vi "Clamp AET Min_Vertical_shan.vi"(0 "Image":T4, 1 "Scanning axis":u16(ring)=1 items=["Left To Right", "Right To Left", "Top To Bottom", "Bottom To Top"], 5 "ROI Descriptor":T5 {"Contours"."Type" items=["No Selection", "Point", "Line", "Rectangle", "Oval", "Polygon", "Freehand Region", "Annulus", "Unused2", "Unused3", "Broken Line", "Freehand Line", "Rotated Rectangle"]}, 7 "Calibrated Image":T4, 9 "Coordinate System":T11 {"Measurement System"."Axis Reference" items=["Direct", "Indirect"]; "Measurement System"."Angle (deg)" format="%.2f"; "Measurement System"."Origin"."Y" format="%.2f"; "Measurement System"."Origin"."X" format="%.2f"; "Reference System"."Axis Reference" items=["Direct", "Indirect"]; "Reference System"."Angle (deg)" format="%.2f"; "Reference System"."Origin"."Y" format="%.2f"; "Reference System"."Origin"."X" format="%.2f"}, 11 "error in (no error)":errorcluster, 12 "Edge Options":T8={"Edge Polarity"=0, "Kernel Size"=3, "Width"=3, "Minimum Edge Strength"=10.0, "Interpolation Type"=enum."Bilinear Fixed", "Data Processing Method"=enum."Average"} {"Edge Polarity" items=["All Edges", "Rising Edges", "Falling Edges"]; "Minimum Edge Strength" format="%.2f"; "Width" step=2; "Kernel Size" step=2}) -> (3 "Edge Coordinates":cluster{"X":sgl, "Y":sgl}[](array[cluster]) {"Y" format="%.2f"; "X" format="%.2f"}, 6 "Distance":sgl format="%.2f", 8 "Coordinate System (duplicate)":T11 {"Measurement System"."Axis Reference" items=["Direct", "Indirect"]; "Measurement System"."Angle (deg)" format="%.2f"; "Measurement System"."Origin"."Y" format="%.2f"; "Measurement System"."Origin"."X" format="%.2f"; "Reference System"."Axis Reference" items=["Direct", "Indirect"]; "Reference System"."Angle (deg)" format="%.2f"; "Reference System"."Origin"."Y" format="%.2f"; "Reference System"."Origin"."X" format="%.2f"}, 10 "Search Lines":T1[](array[typedef]) {"Edge Info"."Distance (Real-World)" format="%.2f"; "Edge Info"."Location (Real-World)"."Y" format="%.2g"; "Edge Info"."Location (Real-World)"."X" format="%.2f"; "Edge Info"."Noise" format="%.2f"; "Edge Info"."Location (Pixel)"."Y" format="%.2g"; "Edge Info"."Location (Pixel)"."X" format="%.2f"; "Edge Info"."Strength" format="%.2f"; "Edge Info"."Distance (Pixel)" format="%.2f"}, 13 "Overlay Cluster out":T3 {"Search Lines"."Edge Info"."Distance (Real-World)" format="%.2f"; "Search Lines"."Edge Info"."Location (Real-World)"."Y" format="%.2g"; "Search Lines"."Edge Info"."Location (Real-World)"."X" format="%.2f"; "Search Lines"."Edge Info"."Noise" format="%.2f"; "Search Lines"."Edge Info"."Location (Pixel)"."Y" format="%.2g"; "Search Lines"."Edge Info"."Location (Pixel)"."X" format="%.2f"; "Search Lines"."Edge Info"."Strength" format="%.2f"; "Search Lines"."Edge Info"."Distance (Pixel)" format="%.2f"}, 14 "Perpendicular Lines":T6(array[cluster])=[{{"X"=55.0, "Y"=48.0}, {"X"=263.0, "Y"=104.0}}, {{"X"=53.0, "Y"=53.0}, {"X"=262.0, "Y"=109.0}}, {{"X"=52.0, "Y"=58.0}, {"X"=261.0, "Y"=113.0}}, {{"X"=51.0, "Y"=62.0}, {"X"=259.0, "Y"=118.0}}, {{"X"=49.0, "Y"=67.0}, {"X"=258.0, "Y"=123.0}}, {{"X"=48.0, "Y"=72.0}, {"X"=257.0, "Y"=128.0}}, {{"X"=47.0, "Y"=77.0}, {"X"=255.0, "Y"=133.0}}, {{"X"=46.0, "Y"=82.0}, {"X"=254.0, "Y"=138.0}}, {{"X"=44.0, "Y"=87.0}, {"X"=253.0, "Y"=142.0}}, {{"X"=43.0, "Y"=91.0}, {"X"=252.0, "Y"=147.0}}, {{"X"=42.0, "Y"=96.0}, {"X"=250.0, "Y"=152.0}}] {"?"."Y" format="%.2f"; "?"."X" format="%.2f"; "?"."Y" format="%.2f"; "?"."X" format="%.2f"}, 15 "error out":errorcluster)   [LabVIEW 2019, in "Algorithm.lvclass"]
doc: "Modified NI Vertical Max Clamp with Rake-3 which uses Advanced Edge Detection."
uses:
  FrameworkOverrides/Algorithm.lvclass
  <vilib>/vision/NI_Vision_Development_Module.lvlib
  <vilib>/vision/Measure.llb/Edge New.ctl
  <vilib>/vision/Measure.llb/Search Line.ctl
  <vilib>/vision/Image Controls.llb/IMAQ Image.ctl
  <vilib>/vision/Measure.llb/Edge Polarity.ctl
  <vilib>/vision/Measure.llb/Edge Options.ctl
panel:
  in  "Rect for the clamp":T7 {"Rotation" format="%.2f"; "Left" scale=0.0..1024.0; "Right" scale=0.0..1024.0}
  in  "Settings":T10={"Contrast"=50, "Filter width"=4, "Steepness"=2, "Subsampling Ratio"=5, "Show Search Area"=FALSE, "Show Search Lines"=FALSE, "Show Edges Found"=FALSE, "Show Result"=TRUE}
  out "Elapsed time (ms)":u32
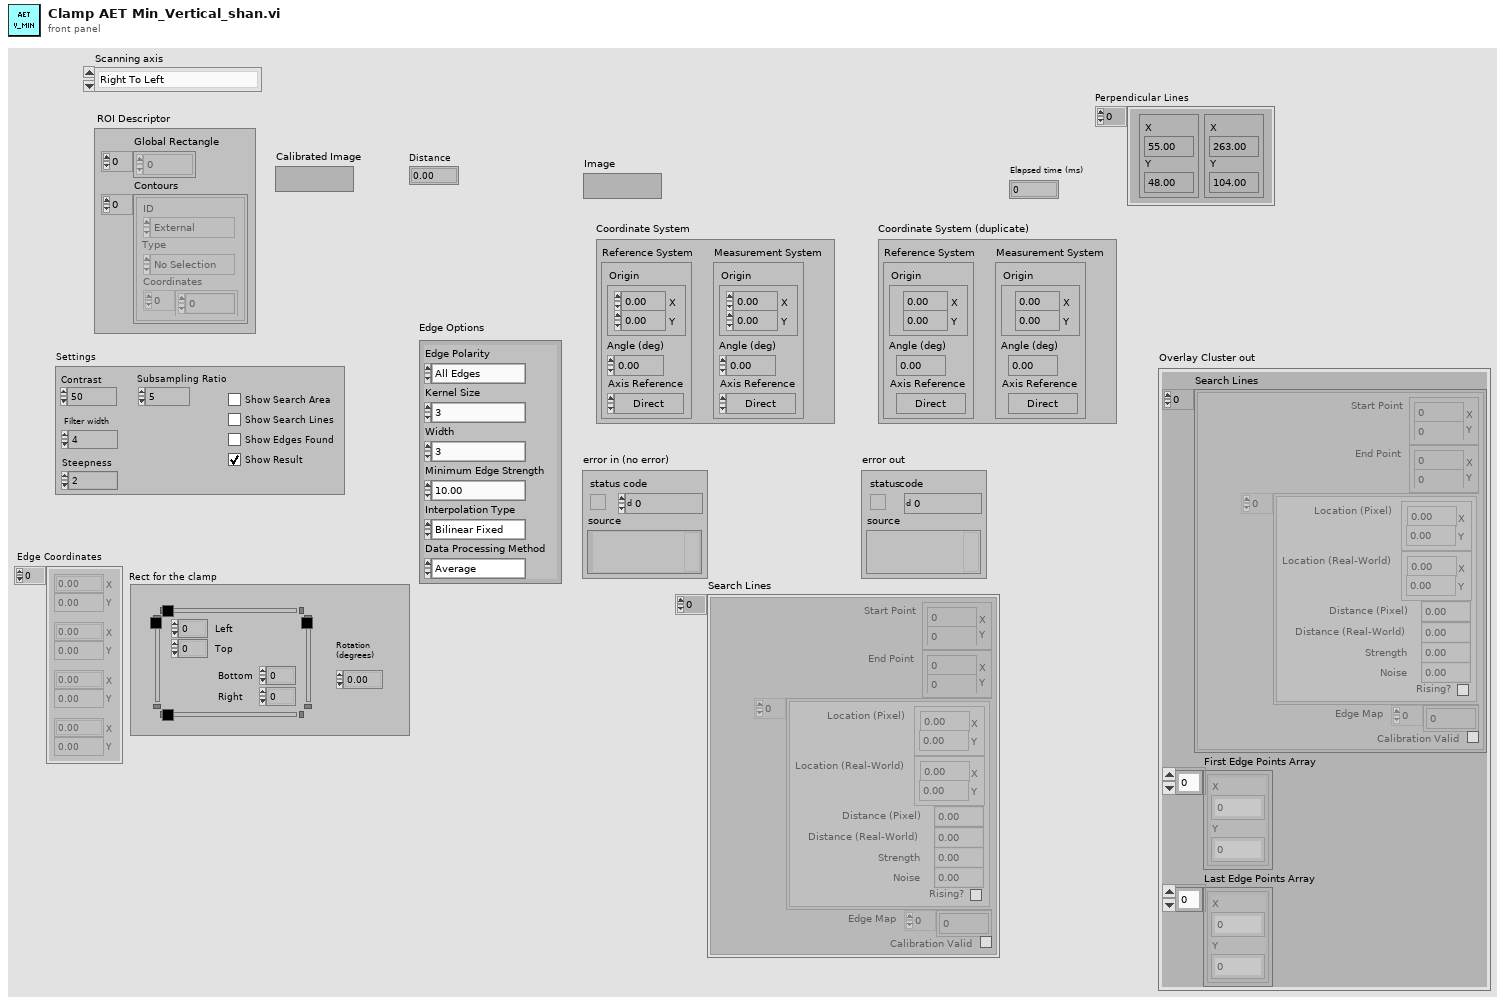
[diagram p1: front panel]
types:
  T1 = typedef "Search Line.ctl" = cluster{"Start Point":cluster{"X":sgl, "Y":sgl}, "End Point":cluster{"X":sgl, "Y":sgl}, "Edge Info":T2[], "Edge Map":dbl[], "Calibration Valid":bool}
  T2 = typedef "Edge New.ctl" = cluster{"Location (Pixel)":cluster{"X":sgl, "Y":sgl}, "Location (Real-World)":cluster{"X":sgl, "Y":sgl}, "Distance (Pixel)":dbl, "Distance (Real-World)":dbl, "Strength":dbl, "Noise":dbl, "Rising?":bool}
  T3 = cluster{"Search Lines":T1[], "First Edge Points Array":cluster{"X":sgl, "Y":sgl}[], "Last Edge Points Array":cluster{"X":sgl, "Y":sgl}[]}
  T4 = typedef "IMAQ Image.ctl" = refnum<image>
  T5 = typedef "ROI Descriptor" = cluster{"Global Rectangle":i32[], "Contours":cluster{"ID":enum32{"External", "Internal"}, "Type":u32, "Coordinates":i32[]}[]}
  T6 = cluster{cluster{"X":sgl, "Y":sgl}, cluster{"X":sgl, "Y":sgl}}[]
  T7 = typedef "IMAQ Rectangle" = cluster{"Left":i32, "Top":i32, "Right":i32, "Bottom":i32, "Rotation":dbl}
  T8 = typedef "Edge Options.ctl" = cluster{"Edge Polarity":T9, "Kernel Size":u32, "Width":u32, "Minimum Edge Strength":sgl, "Interpolation Type":enum32{"Zero Order", "Bilinear", "Quadratic", "Cubic", "Bilinear Fixed"}, "Data Processing Method":enum32{"Average", "Median"}}
  T9 = typedef "Edge Polarity.ctl" = u32
  T10 = cluster{"Contrast":i32, "Filter width":i32, "Steepness":i32, "Subsampling Ratio":u32, "Show Search Area":bool, "Show Search Lines":bool, "Show Edges Found":bool, "Show Result":bool}
  T11 = typedef "IMAQ Coordinate System" = cluster{"Reference System":cluster{"Origin":cluster{"X":sgl, "Y":sgl}, "Angle (deg)":sgl, "Axis Reference":u32}, "Measurement System":cluster{"Origin":cluster{"X":sgl, "Y":sgl}, "Angle (deg)":sgl, "Axis Reference":u32}}
  T12 = enum16{"Get First Edge", "Get First + Last Edge", "Get All Edges", "Get Best Edge"}
  T13 = cluster{"Start Point":cluster{"X":sgl, "Y":sgl}, "End Point":cluster{"X":sgl, "Y":sgl}}
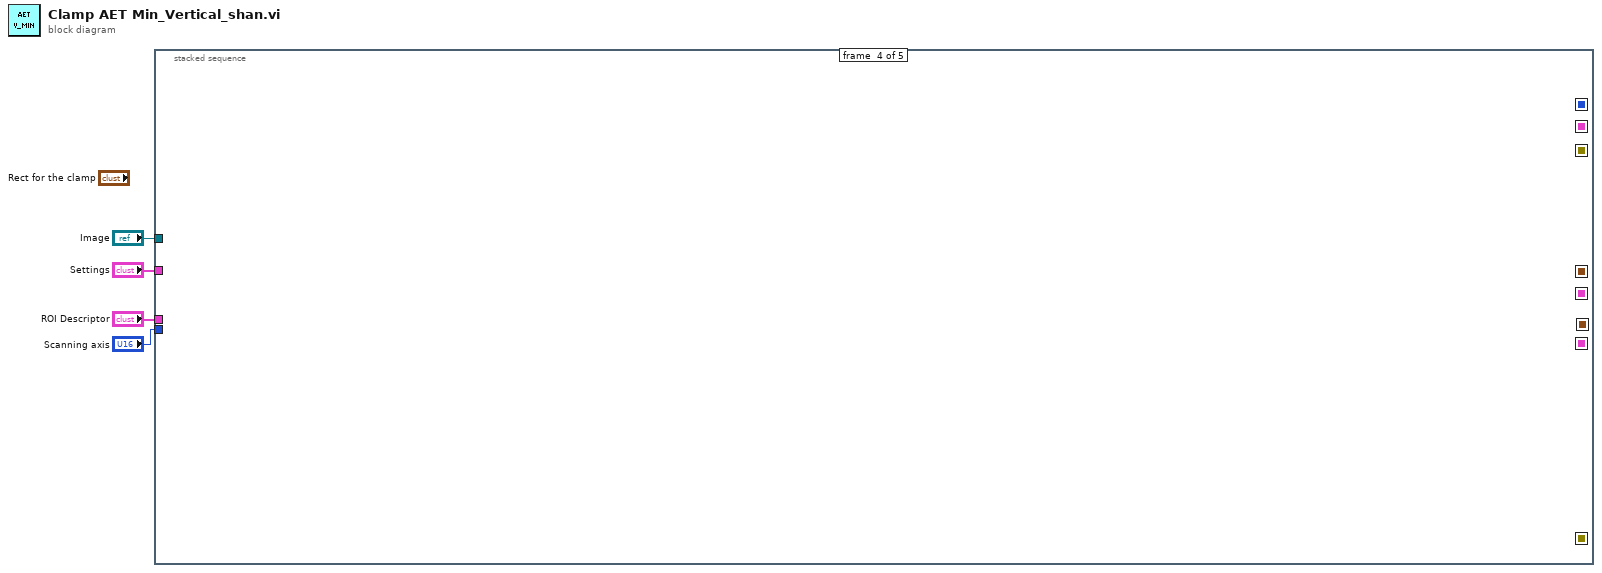
[diagram p0: block diagram]
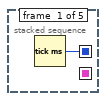
[diagram p2: hidden frame]
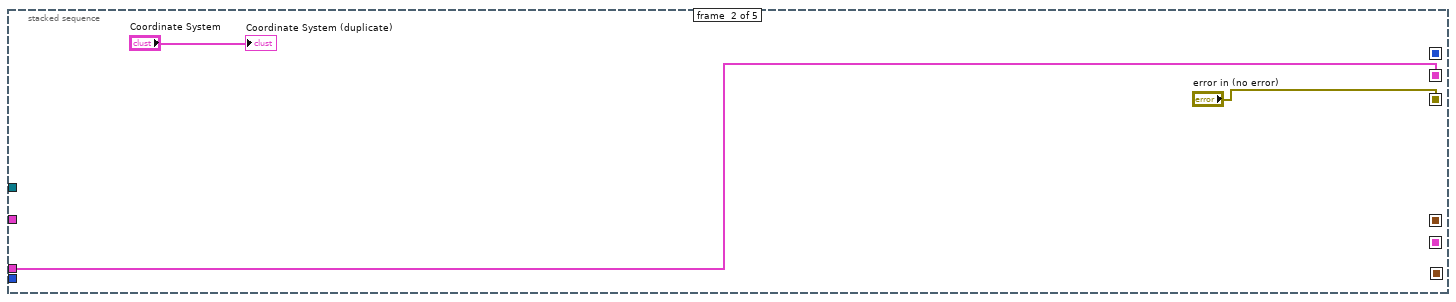
[diagram p3: hidden frame]
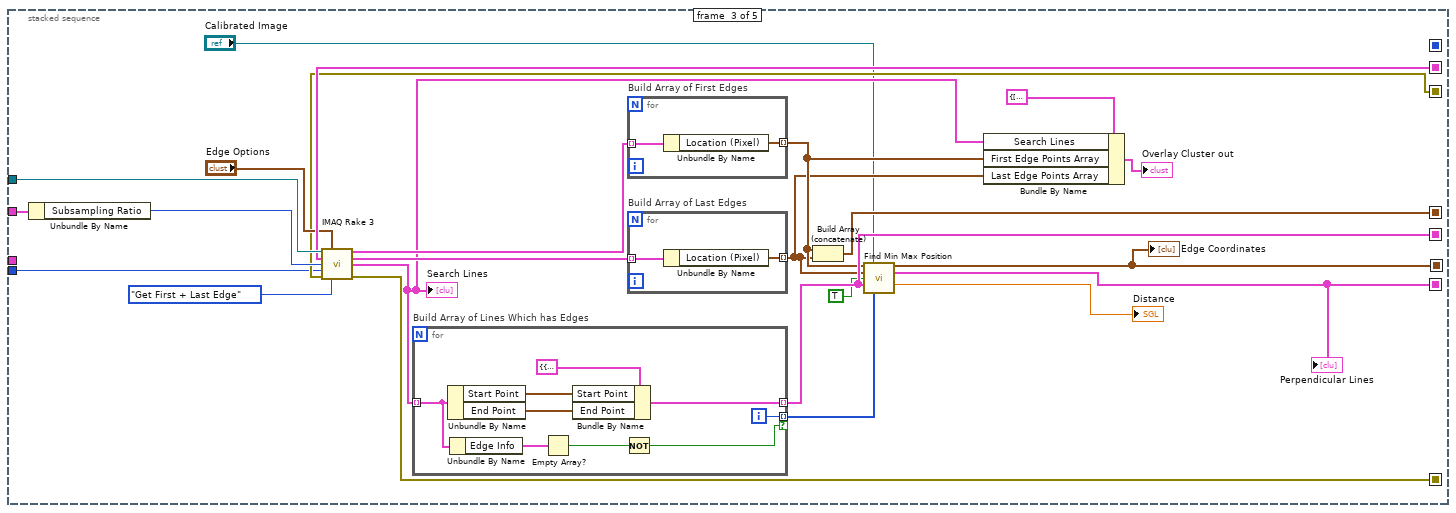
[diagram p4: hidden frame]
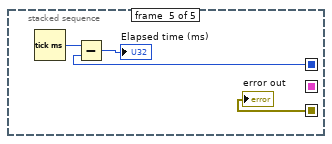
[diagram p5: hidden frame]
diagram:
  n1 = stacked-sequence {
    seq-local: [_ _ w22 _ _] -> [_ _ _ _ _]
    seq-local: [w5 _ _ _ _] -> [_ _ _ _ w49]
    seq-local: [_ _ w24 _ _] -> [_ _ _ _ _]
    seq-local: [_ _ w25 _ _] -> [_ _ _ _ _]
    seq-local: [_ _ w23 _ _] -> [_ _ _ _ _]
    seq-local: [_ w6 _ _ _] -> [_ _ w30 _ _]
    seq-local: [_ "error in (no error)" _ _ _] -> [_ _ w18 _ w46]
    seq-local: [_ _ w17 _ _] -> [_ _ _ _ _]
    tunnel: "Image" -> [_ _ w31 _ _]
    tunnel: "Settings" -> [_ _ w32 _ _]
    tunnel: "ROI Descriptor" -> [_ w6 _ _ _]
    tunnel: "Scanning axis" -> [_ _ w15 _ _]
    frame #0 {
      n2 = Tick Count (ms)() -> (millisecond timer value=w5:u32)
    }
    frame #1 {
      "Coordinate System (duplicate)" <- "Coordinate System"
    }
    frame #2 {
      n3 = Unbundle By Name(w32) -> ("Subsampling Ratio"=w29:u32)
      n4 = call "IMAQ Rake 3"("Image"=w31, "Edge Options"="Edge Options", "ROI Descriptor"=w30, "Step Size"=w29, "Scan Direction"=w15, "error in (no error)"=w18, "Process"=T12."Get First + Last Edge") -> ("First Edges"=w27:T2[], "Last Edges"=w26:T2[], "Search Lines"=w13:T1[], "error out"=w17:errorcluster)  [unwired: 5 in]
      "Search Lines" <- w13
      n5 = for "Build Array of Lines Which has Edges" {
        tunnel: w13 -> [w38] mode=indexing
        tunnel: [w39] -> w25 mode=indexing
        tunnel: [w35] -> w20 mode=indexing if=w34
        i -> [w35]
        n6 = Unbundle By Name(w38) -> ("Start Point"=w41:cluster{"X":sgl, "Y":sgl}, "End Point"=w40:cluster{"X":sgl, "Y":sgl})
        n7 = Unbundle By Name(w38) -> ("Edge Info"=w37:T2[])
        n8 = Empty Array?(array=w37) -> (empty?=w36:bool)
        n9 = Bundle By Name(cluster=T13 {"Start Point"={"X"=0.0, "Y"=0.0}, "End Point"={"X"=0.0, "Y"=0.0}} ("Cluster 2"), "Start Point"=w41, "End Point"=w40) -> (w39:T13)
        n10 = Not(x=w36) -> (.not. x?=w34:bool)
      }
      n11 = for "Build Array of First Edges" {
        tunnel: w27 -> [w45] mode=indexing
        tunnel: [w44] -> w12 mode=indexing
        n12 = Unbundle By Name(w45) -> ("Location (Pixel)"=w44:cluster{"X":sgl, "Y":sgl})
      }
      n13 = for "Build Array of Last Edges" {
        tunnel: w26 -> [w43] mode=indexing
        tunnel: [w42] -> w11 mode=indexing
        n14 = Unbundle By Name(w43) -> ("Location (Pixel)"=w42:cluster{"X":sgl, "Y":sgl})
      }
      n15 = Build Array (concatenate)(w12, w11) -> (w24:cluster{"X":sgl, "Y":sgl}[])
      n16 = call "Find Min Max Position.vi"("First Edges"=w12, "Calibrated Image"="Calibrated Image", "Last Edges"=w11, "Min / Max"=TRUE, "Search Lines"=w25, "Lines with Edges (first)"=w20) -> ("Points"=w22:cluster{"X":sgl, "Y":sgl}[], "Perpendicular Lines"=w23:T6, "Distance"=→"Distance":sgl)  [unwired: 6 in, 1 out]
      "Edge Coordinates" <- w22
      "Perpendicular Lines" <- w23
      n17 = Bundle By Name(cluster=T3 {"Search Lines"=[], "First Edge Points Array"=[], "Last Edge Points Array"=[]} ("Overlay Cluster out"), "Search Lines"=w13, "First Edge Points Array"=w12, "Last Edge Points Array"=w11) -> (→"Overlay Cluster out":T3)
    }
    frame #3 {
    }
    frame #4 {
      n18 = Tick Count (ms)() -> (millisecond timer value=w48:u32)
      n19 = Subtract(x=w48, y=w49) -> (x-y=→"Elapsed time (ms)":u32)
      "error out" <- w46
    }
  }
